vi "Config Config to String.vi"(8 "error in":errorcluster, 11 "Config Cluster in":T1) -> (0 "error out":errorcluster, 3 "Output String":string)   [LabVIEW 2017]
uses:
  Config Cluster.ctl
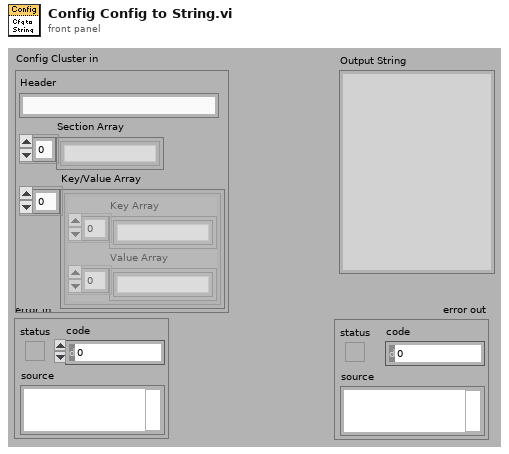
[diagram p1: front panel]
types:
  T1 = typedef "Config Cluster.ctl" = cluster{"Header":string, "Section Array":string[], "Key/Value Array":cluster{"Key Array":string[], "Value Array":string[]}[]}
  T2 = cluster{"Key Array":string[], "Value Array":string[]}[]
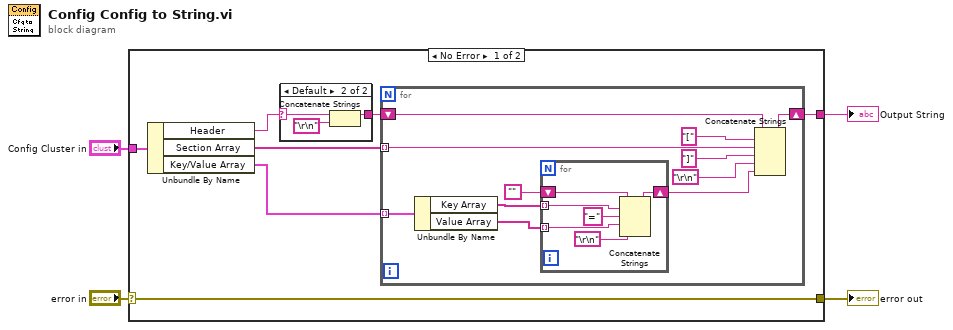
[diagram p0: block diagram]
diagram:
  n1 = case shown="No Error" "error in" {
    selector: "error in" -> [w7 w33]
    tunnel: [w7 w33] -> w3
    tunnel: "Config Cluster in" -> [w9 _]
    tunnel: [w8 _] -> w1
    frame No Error {
      n2 = Unbundle By Name(w9) -> ("Header"=w5:string, "Section Array"=w11:string[], "Key/Value Array"=w10:T2)
      n3 = case shown="Default" w5 {
        selector: w5 -> [w12 w14]
        tunnel: [w12 w15] -> w6
        frame "" {
        }
        frame Default {
          n4 = Concatenate Strings(w14, "\r\n") -> (w15:string)
        }
      }
      n5 = for {
        tunnel: w11 -> [w25] mode=indexing
        tunnel: w10 -> [w26] mode=indexing
        shift-right: [w22] -> w8
        shift-left: w6 -> [w17]
        n6 = Unbundle By Name(w26) -> ("Key Array"=w21:string[], "Value Array"=w20:string[])
        n7 = for {
          tunnel: w21 -> [w32] mode=indexing
          tunnel: w20 -> [w30] mode=indexing
          shift-right: [w29] -> w18
          shift-left: "" -> [w28]
          n8 = Concatenate Strings(w28, w32, "=", w30, "\r\n") -> (w29:string)
        }
        n9 = Concatenate Strings(w17, "[", w25, "]", "\r\n", w18) -> (w22:string)
      }
    }
    frame Error {
    }
  }
  "error out" <- w3
  "Output String" <- w1
